vi "ReadWaveDataProcess.vi"(8 "error in (no error)":errorcluster, 11 "ScopeBB in":refnum<class "ScopeBB.lvclass">) -> (0 "error out":errorcluster, 2 "Waveform":waveform(dbl), 3 "ScopeBB out":refnum<class "ScopeBB.lvclass">)   [LabVIEW 2018, in "ScopeBB.lvclass"]
uses:
  ScopeBB.lvclass
  <vilib>/measure/NI_MABase.lvlib
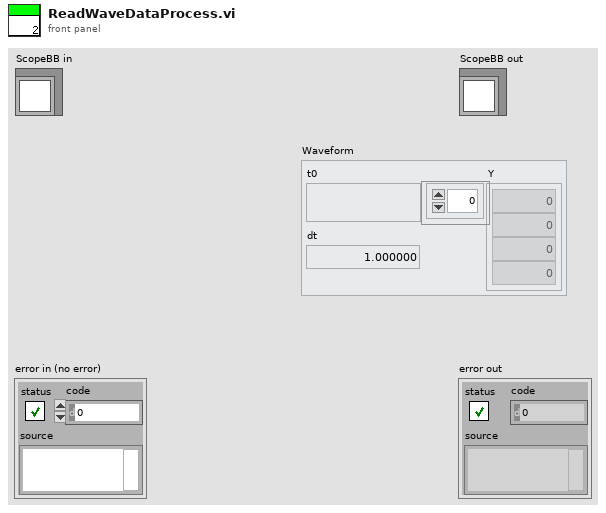
[diagram p1: front panel]
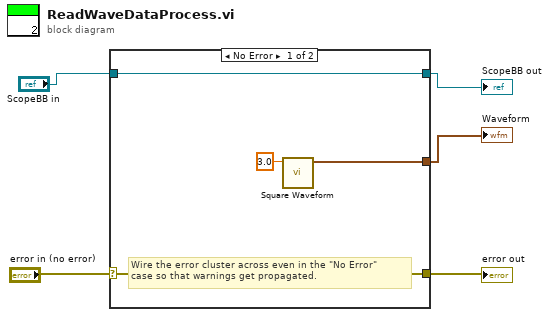
[diagram p0: block diagram]
diagram:
  n1 = case shown="No Error" "error in (no error)" {
    selector: "error in (no error)" -> [w8 w11]
    tunnel: [w8 w11] -> w1
    tunnel: [w9 w10] -> w4
    tunnel: "ScopeBB in" -> [w9 w10]
    tunnel: [w7 _] -> w3
    frame No Error {
      # "Wire the error cluster across even in the \"No Error\"\ncase so that warnings get propagated."
      n2 = call <vilib>:"Square Waveform.vi"("frequency"=3.0) -> ("signal out"=w7:waveform(dbl))  [unwired: 9 in, 1 out]
    }
    frame Error {
    }
  }
  "error out" <- w1
  "ScopeBB out" <- w4
  "Waveform" <- w3
